vi "Reset NIC.vi"(8 "Error In":errorcluster, 10 "NIC Name":string, 11 "Install LV Data":T1) -> (0 "Error Out":errorcluster, 3 "Install LV Data out":T1)   [LabVIEW 2020, in "LMH-LINX.lvlib"]
uses:
  LMH-LINX.lvlib
  Install LV Data.ctl
  Target Info.ctl
  NIC Info.ctl
  NIC Mode.ctl
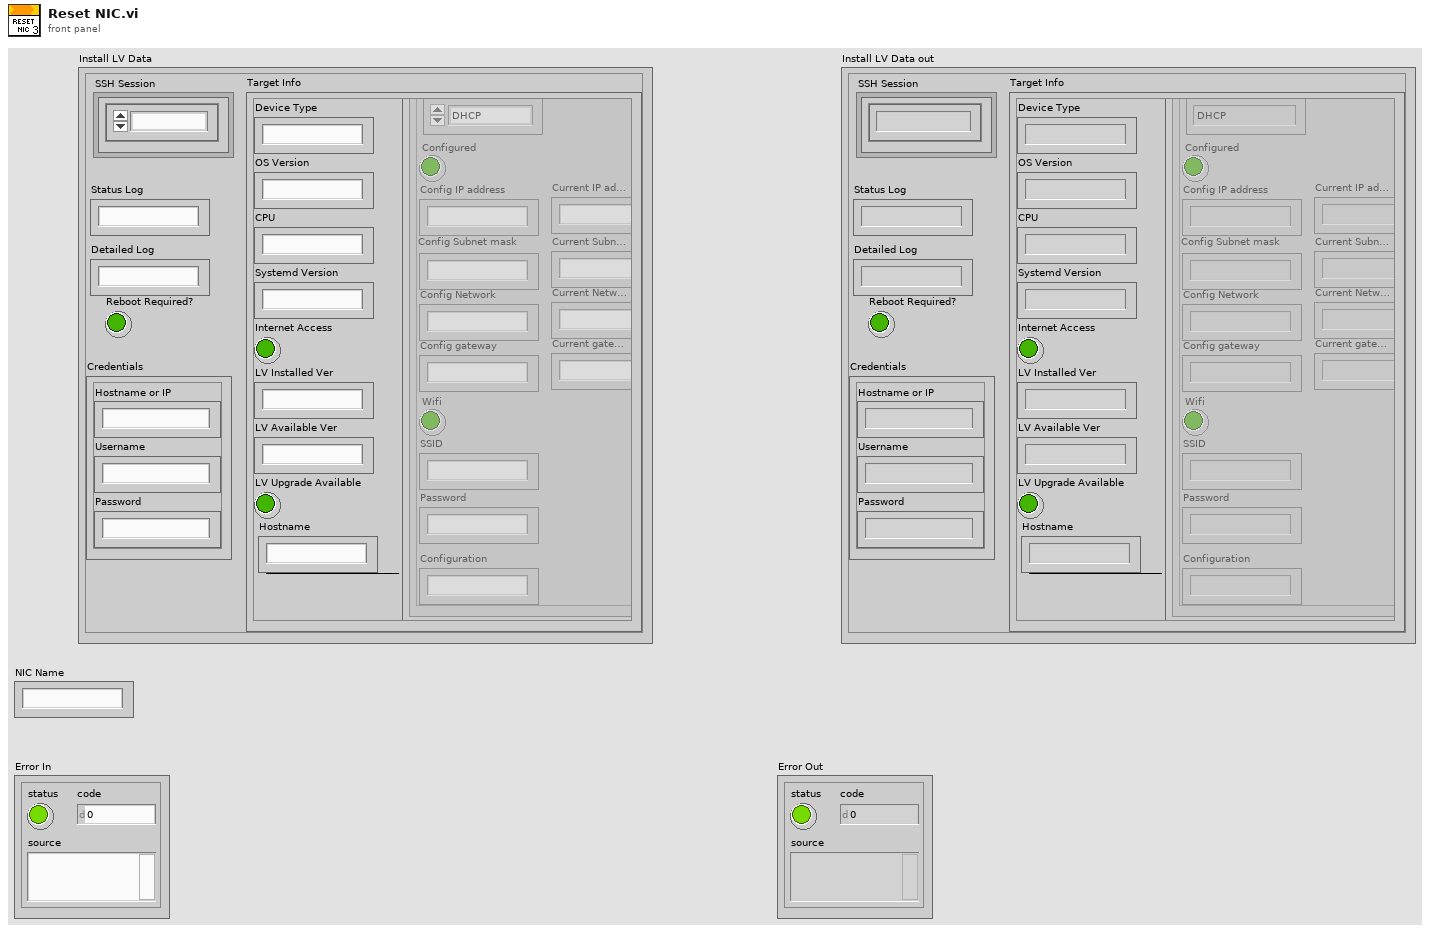
[diagram p1: front panel]
types:
  T1 = typedef "LMH-LINX.lvlib/Install LV Data.ctl" = cluster{"SSH Session":refnum<k1>, "Status Log":string, "Detailed Log":string, "Credentials":cluster{"Hostname or IP":string, "Username":string, "Password":string}, "Target Info":T2, "Reboot Required?":bool}
  T2 = typedef "LMH-LINX.lvlib/Target Info.ctl" = cluster{"OS Version":string, "CPU":string, "Systemd Version":string, "Internet Access":bool, "Device Type":string, "LV Installed Ver":string, "LV Available Ver":string, "LV Upgrade Available":bool, "Hostname":string, "NIC Info":T3[]}
  T3 = typedef "LMH-LINX.lvlib/NIC Info.ctl" = cluster{"Name":string, "NIC Mode":T4, "Configured":bool, "Config IP address":string, "Config Subnet mask":string, "Config Network":string, "Config gateway":string, "Wifi":bool, "SSID":string, "Password":string, "Configuration":string, "Current IP address":string, "Current Subnet mask":string, "Current gateway":string, "Current Network":string}
  T4 = typedef "LMH-LINX.lvlib/NIC Mode.ctl" = enum16{"DHCP", "Static", "Loopback"}
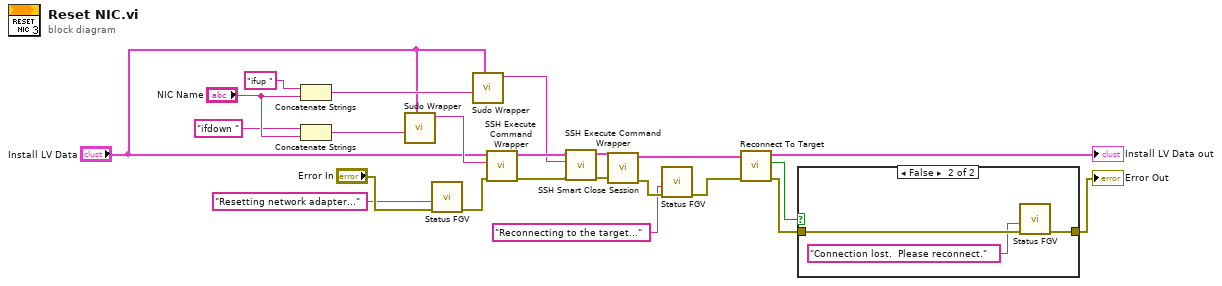
[diagram p0: block diagram]
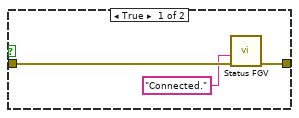
[diagram p2: hidden frame]
diagram:
  n1 = Concatenate Strings("ifup " ("string"), "NIC Name") -> (w3:string)
  n2 = Concatenate Strings("ifdown " ("string"), "NIC Name") -> (w6:string)
  n3 = call "Sudo Wrapper.vi"("Install LV Data"="Install LV Data", "comand string"=w6) -> ("combined command string"=w5:string)  [unwired: 9 in]
  n4 = call "Status FGV.vi"("Error In"="Error In", "Status"="Resetting network adapter...") -> ("Error Out"=w20:errorcluster)  [unwired: 7 in, 2 out]
  n5 = call "Sudo Wrapper.vi"("Install LV Data"="Install LV Data", "comand string"=w3) -> ("combined command string"=w2:string)  [unwired: 9 in]
  n6 = call "SSH Execute Command Wrapper.vi"("Error In"=w20, "Command"=w5, "Install LV Data in"="Install LV Data") -> ("Error Out"=w9:errorcluster, "Install LV Data out"=w8:T1)  [unwired: 6 in, 1 out]
  n7 = call "SSH Execute Command Wrapper.vi"("Error In"=w9, "Command"=w2, "Install LV Data in"=w8) -> ("Error Out"=w10:errorcluster, "Install LV Data out"=w11:T1)  [unwired: 6 in, 1 out]
  n8 = call "SSH Smart Close Session.vi"("Error In"=w10, "Install LV Data"=w11) -> ("Error Out"=w18:errorcluster, "Install LV Data"=w17:T1)  [unwired: 8 in]
  n9 = call "Status FGV.vi"("Error In"=w18, "Status"="Reconnecting to the target...") -> ("Error Out"=w16:errorcluster)  [unwired: 7 in, 2 out]
  n10 = call "Reconnect To Target.vi"("Error In"=w16, "Install LV Data in"=w17) -> ("Error Out"=w14:errorcluster, "Connected?"=w12:bool, "Install LV Data out"=→"Install LV Data out":T1)  [unwired: 7 in]
  n11 = case shown="False" w12 {
    tunnel: w14 -> [w26 w29]
    tunnel: [w25 w28] -> w13
    frame True {
      n12 = call "Status FGV.vi"("Error In"=w26, "Status"="Connected.") -> ("Error Out"=w25:errorcluster)  [unwired: 7 in, 2 out]
    }
    frame False {
      n13 = call "Status FGV.vi"("Error In"=w29, "Status"="Connection lost.  Please reconnect.") -> ("Error Out"=w28:errorcluster)  [unwired: 7 in, 2 out]
    }
  }
  "Error Out" <- w13
